vi "FGV_DOCK_error_buffer.vi"(4 "main_tab":refnum<vi>, 6 "thread":T1, 7 "option":T2=enum."display", 8 "error_in":errorcluster, 9 "error_indicator_global":refnum<vi>, 10 "error_indicator_tab":refnum<vi>, 11 "error_display_ref":refnum<vi>) -> (0 "error_out":errorcluster, 3 "error?":bool)   [LabVIEW 2019]
doc: "This VI check if error on error_in input is already in the buffer, and if not adds it to buffer and sends error event to event structure. VI also clears errors."
uses:
  FGV_DOCK_error_buffer.ctl
  MAIN/DOCK_thread.ctl
  <vilib>/Utility/miscctls.llb/LVRowAndColumnTypeDef.ctl
  <vilib>/Utility/miscctls.llb/LVRowAndColumnUnsignedTypeDef.ctl
  DOCK_multistate_indicator/FGV_DOCK_multistate_indicator.ctl
  _misc/AULocalize/SubVIs/Get Localized Phrase Compact Interface 1D.vi
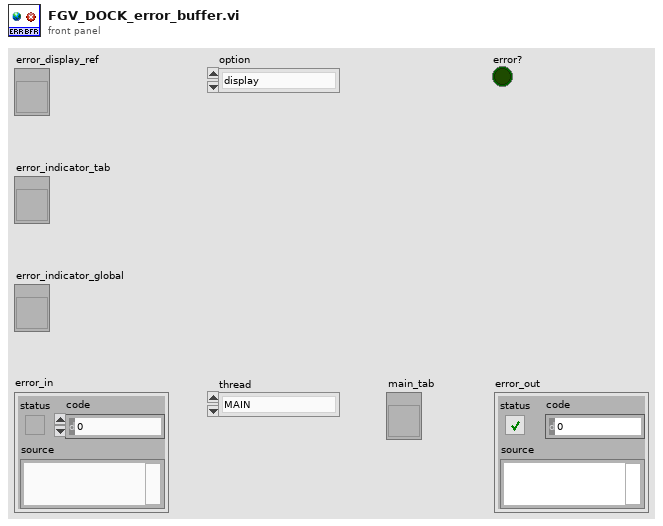
[diagram p1: front panel]
types:
  T1 = typedef "DOCK_thread.ctl" = enum16{"MAIN", "SCANNER", "PRINTER"}
  T2 = typedef "FGV_DOCK_error_buffer.ctl" = enum16{"initialize", "clear", "display", "get_status"}
  T3 = typedef "LVRowAndColumnUnsignedTypeDef.ctl" = cluster{"Row":u32, "Column":u32}
  T4 = typedef "LVRowAndColumnTypeDef.ctl" = cluster{"Row":i32, "Column":i32}
  T5 = typedef "FGV_DOCK_multistate_indicator.ctl" = enum16{"initialize", "login", "logout", "start_batch", "finish_batch", "gear_OK", "gear_NOK", "gear_clear", "translate", "error", "error_clear"}
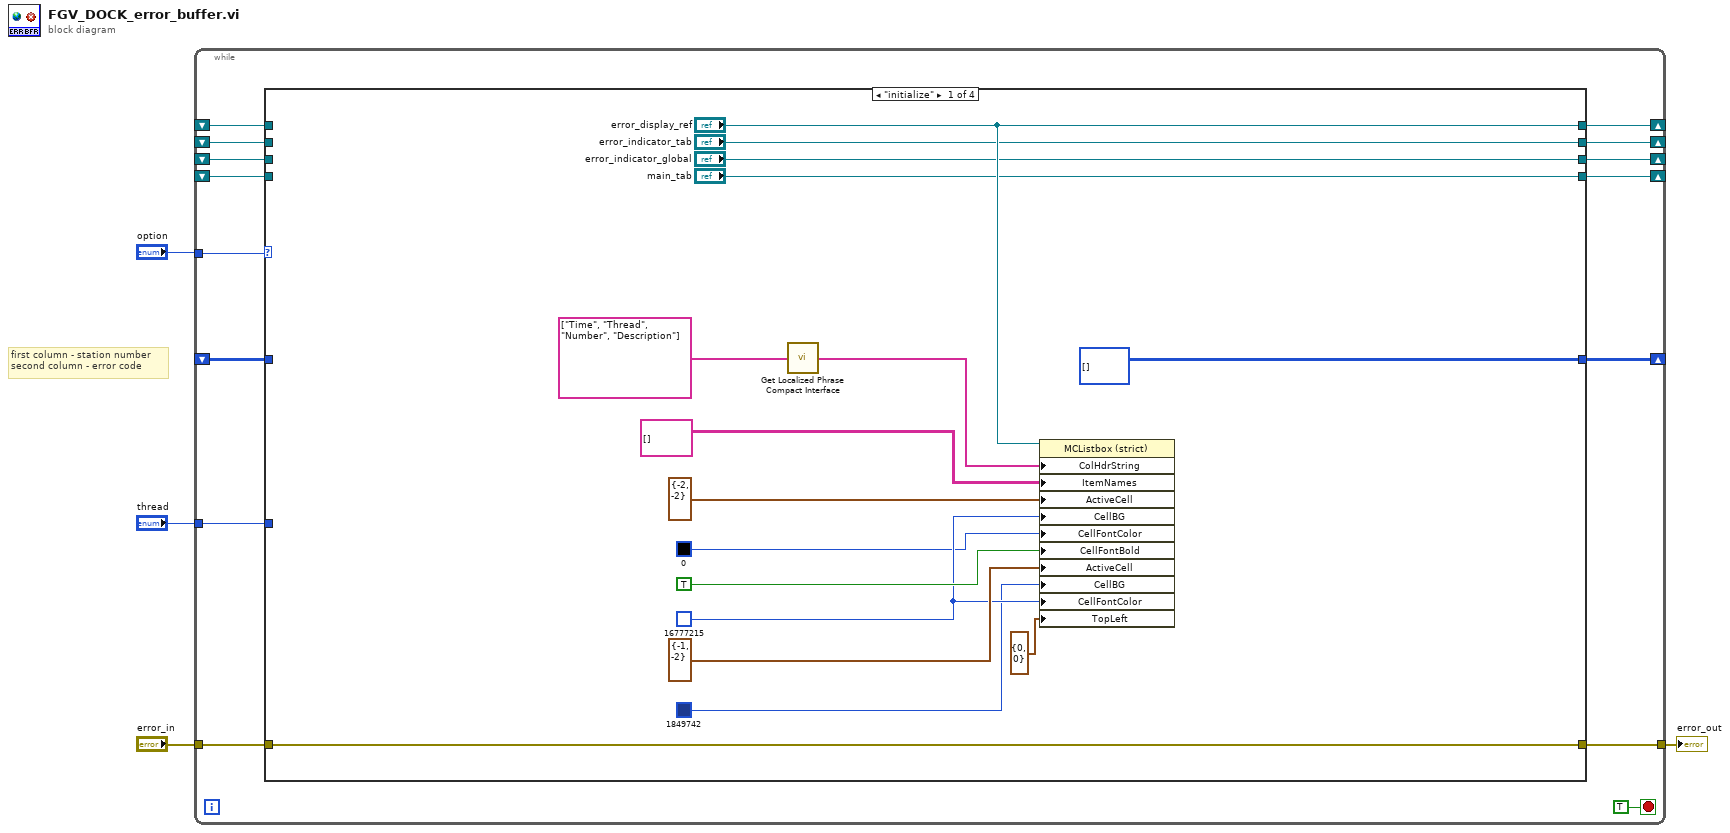
[diagram p0: block diagram]
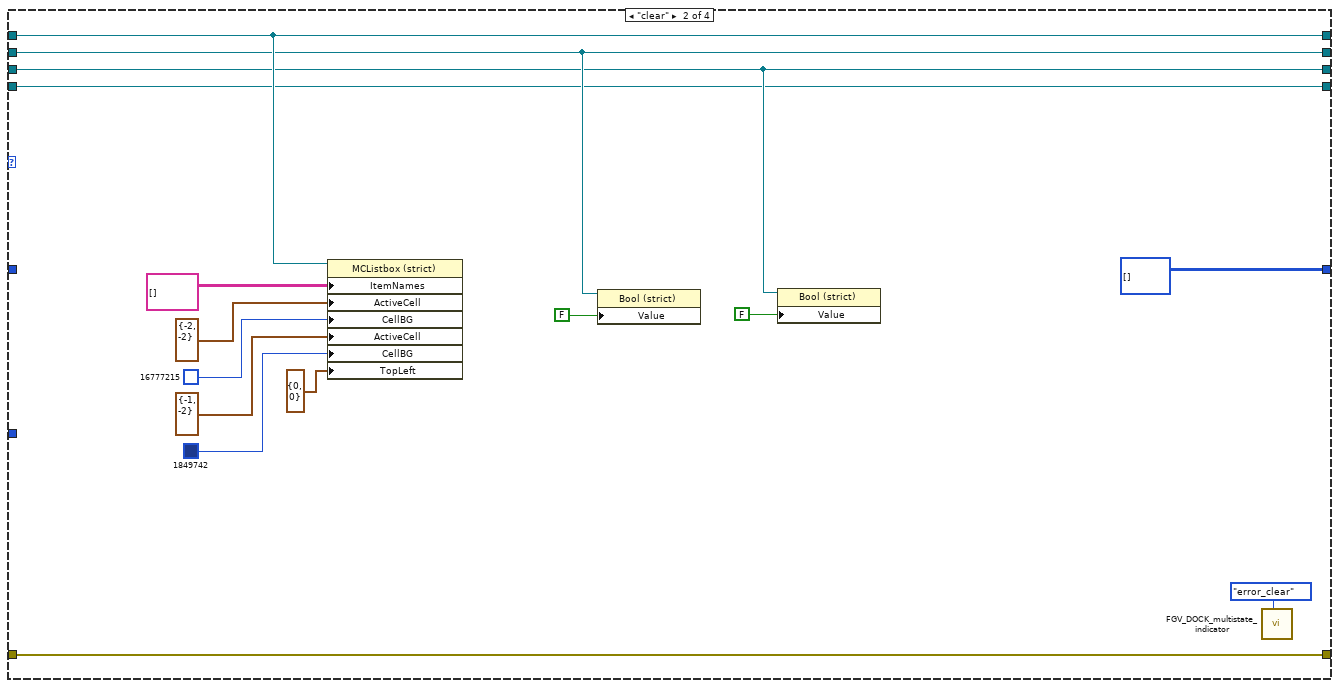
[diagram p2: hidden frame]
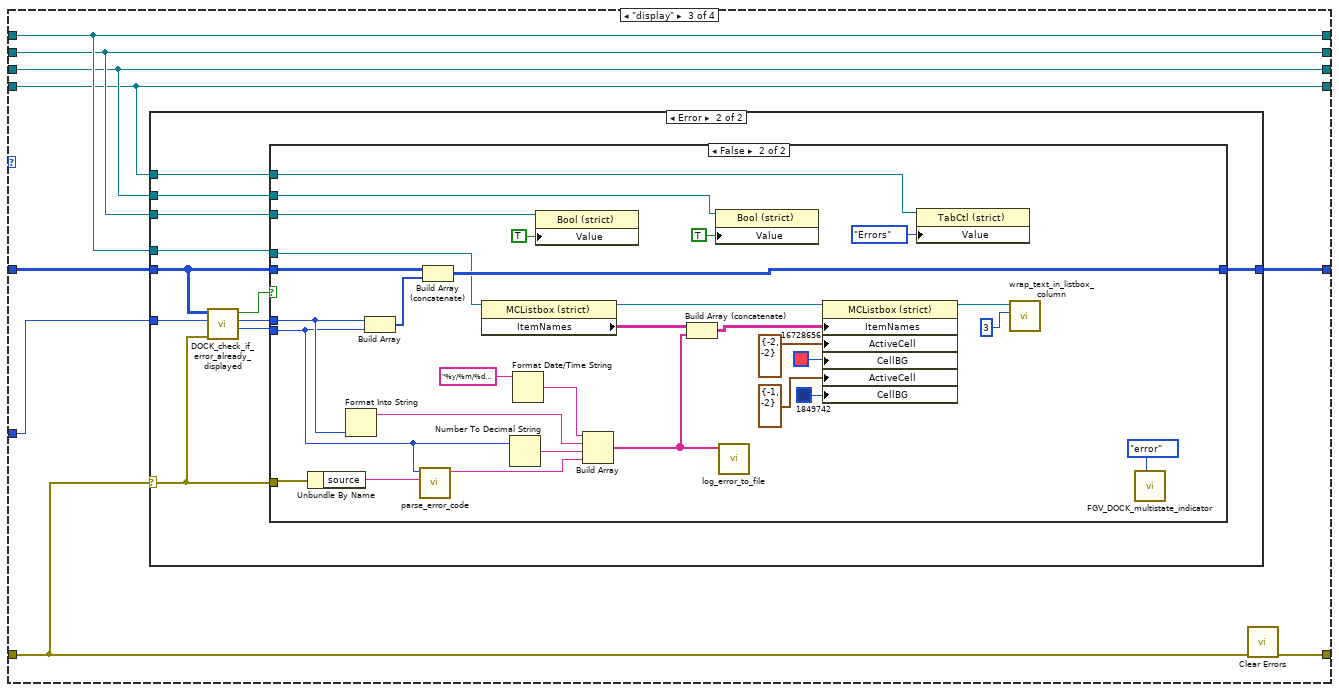
[diagram p3: hidden frame]
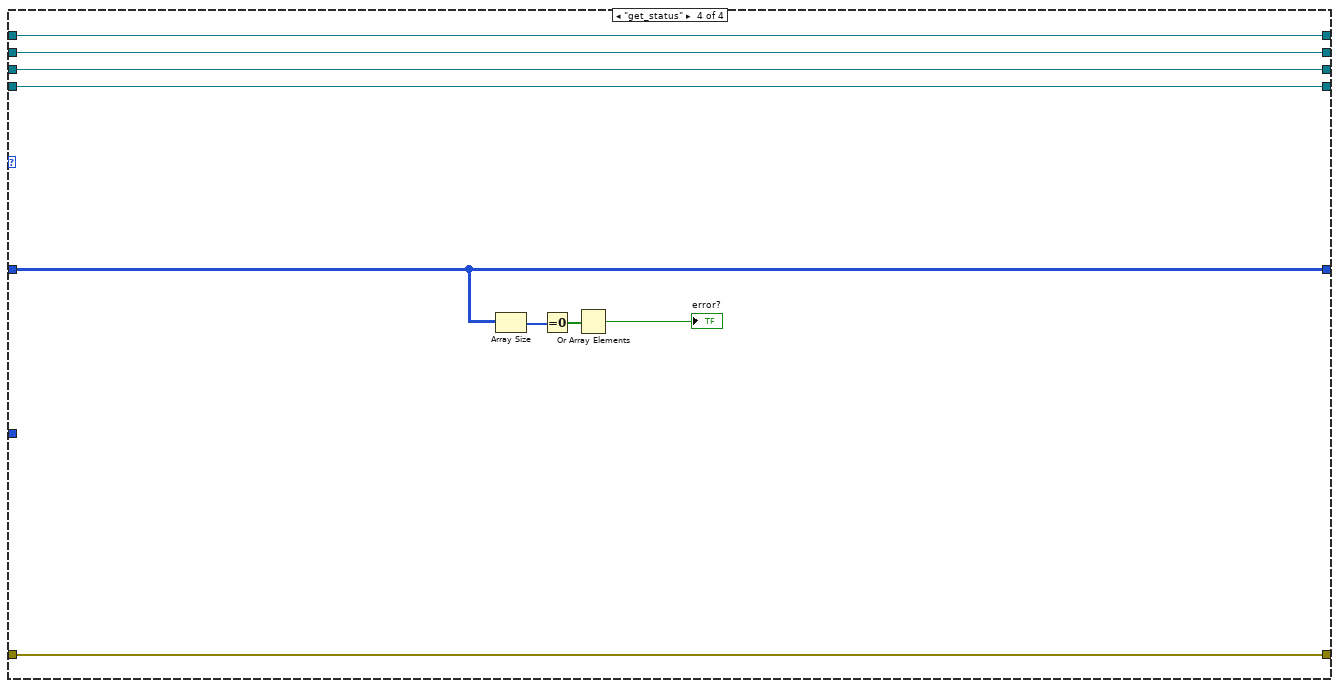
[diagram p6: hidden frame]
diagram:
  # "first column - station number\nsecond column - error code"
  n1 = while {
    tunnel: "option" -> [w18]
    tunnel: [w17] -> w4
    tunnel: "error_in" -> [w16]
    shift-right: [w15] -> _
    shift-left: _ -> [w14]
    shift-right: [w13] -> _
    shift-left: _ -> [w12]
    tunnel: "thread" -> [w11]
    shift-right: [w10] -> _
    shift-left: _ -> [w8]
    shift-right: [w9] -> _
    shift-left: _ -> [w7]
    shift-right: [w6] -> _
    shift-left: _ -> [w5]
    stop <- TRUE stop-if-true
    n2 = case shown="\"initialize\"" w18 {
      tunnel: [w35 w50 w58 w110] -> w17
      tunnel: w16 -> [w35 w50 w57 w110]
      tunnel: [i32[][] [] i32[][] [] w56 w111] -> w15
      tunnel: w14 -> [_ _ w59 w111]
      tunnel: ["error_display_ref" w43 w54 w109] -> w13
      tunnel: w12 -> [_ w43 w54 w109]
      tunnel: w11 -> [_ _ w55 _]
      tunnel: ["error_indicator_tab" w42 w53 w105] -> w10
      tunnel: ["error_indicator_global" w41 w52 w104] -> w9
      tunnel: w8 -> [_ w42 w53 w105]
      tunnel: w7 -> [_ w41 w52 w104]
      tunnel: ["main_tab" w38 w51 w103] -> w6
      tunnel: w5 -> [_ w38 w51 w103]
      frame "initialize" {
        w31 = u32 16777215
        n3 = call-poly "Get Localized Phrase Compact Interface.vi"("Key"=string[] ["Time", "Thread", "Number", "Description"] ("Column Header Strings[]")) -> ("Translated Phrase"=w20:string[])
        n4 = property on="Property Node" class="MCListbox (strict)"(reference="error_display_ref", "ColHdrString"=w20, "ItemNames"=string[][] [] ("Item Names"), "ActiveCell"=T4 {"Row"=-2, "Column"=-2} ("Active Cell:Active Cell"), "CellBG"=w31, "CellFontColor"=u32 0, "CellFontBold"=TRUE ("Active Cell:Cell Font:Bold"), "ActiveCell"=T4 {"Row"=-1, "Column"=-2} ("Active Cell:Active Cell"), "CellBG"=u32 1849742, "CellFontColor"=w31, "TopLeft"=T3 {"Row"=0, "Column"=0} ("Top Left Visible Cell")) -> ()  [unwired: 1 in, 2 out]
      }
      frame "clear" {
        n5 = property on="Property Node" class="MCListbox (strict)"(reference=w43, "ItemNames"=string[][] [] ("Item Names"), "ActiveCell"=T4 {"Row"=-2, "Column"=-2} ("Active Cell:Active Cell"), "CellBG"=u32 16777215, "ActiveCell"=T4 {"Row"=-1, "Column"=-2} ("Active Cell:Active Cell"), "CellBG"=u32 1849742, "TopLeft"=T3 {"Row"=0, "Column"=0} ("Top Left Visible Cell")) -> ()  [unwired: 1 in, 2 out]
        n6 = property on="Property Node" class="Bool (strict)"(reference=w42, "Value"=FALSE) -> ()  [unwired: 1 in, 2 out]
        n7 = property on="Property Node" class="Bool (strict)"(reference=w41, "Value"=FALSE) -> ()  [unwired: 1 in, 2 out]
        n8 = call "FGV_DOCK_multistate_indicator.vi"("options"=FGV_DOCK_multistate_indicator."error_clear") -> ()  [unwired: 10 in, 1 out]
      }
      frame "display" {
        n9 = case shown="Error" w57 {
          selector: w57 -> [_ w65]
          tunnel: w59 -> [w60 w68]
          tunnel: [w60 w70] -> w56
          tunnel: w55 -> [_ w61]
          tunnel: w54 -> [_ w66]
          tunnel: w53 -> [_ w64]
          tunnel: w52 -> [_ w63]
          tunnel: w51 -> [_ w62]
          frame No Error {
          }
          frame Error {
            n10 = call "DOCK_check_if_error_already_displayed.vi"("error_in"=w65, "thread_in"=w61, "displayed_errors"=w68) -> ("error_code"=w67:i32, "thread_out"=w69:T1, "already_displayed?"=w71:bool)  [unwired: 6 in]
            n11 = case shown="False" w71 {
              tunnel: w68 -> [w72 w101]
              tunnel: [w72 w102] -> w70
              tunnel: w69 -> [_ w95]
              tunnel: w67 -> [_ w84]
              tunnel: w66 -> [_ w99]
              tunnel: w65 -> [_ w93]
              tunnel: w64 -> [_ w79]
              tunnel: w63 -> [_ w78]
              tunnel: w62 -> [_ w75]
              frame True {
              }
              frame False {
                n12 = Unbundle By Name(w93) -> ("source"=w85:string)
                n13 = Format Into String(w95) -> (resulting string=w94:string)  [unwired: 3 in, 1 out]
                n14 = Build Array(w95, w84) -> (w100:i32[])
                n15 = call "parse_error_code.vi"("source"=w85, "code"=w84) -> ("parsed_error_string"=w83:string)  [unwired: 9 in]
                n16 = Build Array (concatenate)(w101, w100) -> (w102:i32[][])
                n17 = property class="MCListbox (strict)"(reference=w99) -> (reference out=w87:refnum<vi>, "ItemNames"=w92:string[][])  [unwired: 1 in, 1 out]
                n18 = Number To Decimal String(number=w84) -> (decimal integer string=w96:string)  [unwired: 1 in]
                n19 = Format Date/Time String(time format string (%c)="%y/%m/%d %H:%M:%S") -> (date/time string=w98:string)  [unwired: 2 in]
                n20 = property on="Property Node" class="Bool (strict)"(reference=w79, "Value"=TRUE) -> ()  [unwired: 1 in, 2 out]
                n21 = Build Array(w98, w94, w96, w83) -> (w82:string[])
                n22 = Build Array (concatenate)(w92, w82) -> (w86:string[][])
                n23 = property on="Property Node" class="Bool (strict)"(reference=w78, "Value"=TRUE) -> ()  [unwired: 1 in, 2 out]
                n24 = call "log_error_to_file.vi"("error_info"=w82) -> ()  [unwired: 11 in]
                n25 = property on="Property Node" class="MCListbox (strict)"(reference=w87, "ItemNames"=w86, "ActiveCell"=T4 {"Row"=-2, "Column"=-2} ("Active Cell:Active Cell"), "CellBG"=u32 16728656 ("Color Box"), "ActiveCell"=T4 {"Row"=-1, "Column"=-2} ("Active Cell:Active Cell"), "CellBG"=u32 1849742) -> (reference out=w77:refnum<vi>)  [unwired: 1 in, 1 out]
                n26 = property on="Property Node" class="TabCtl (strict)"(reference=w75, "Value"=enum32{"Dock Audit", "Current Batch", "Errors"}."Errors") -> ()  [unwired: 1 in, 2 out]
                n27 = call "wrap_text_in_listbox_column.vi"("colum_to_wrap"=3, "multicolumn_listbox_reference"=w77) -> ()  [unwired: 8 in, 2 out]
                n28 = call "FGV_DOCK_multistate_indicator.vi"("options"=FGV_DOCK_multistate_indicator."error") -> ()  [unwired: 10 in, 1 out]
              }
            }
          }
        }
        n29 = call <vilib>:"Clear Errors.vi"("error in (no error)"=w57) -> ("error out"=w58:errorcluster)  [unwired: 5 in, 1 out]
      }
      frame "get_status" {
        n30 = Array Size(array=w111) -> (size(s)=w108:i32[])
        n31 = Equal To 0?(x=w108) -> (x = 0?=w107:bool[])
        n32 = Or Array Elements(Boolean array=w107) -> (logical OR=→"error?":bool)
      }
    }
  }
  "error_out" <- w4
